vi "Get_CtrFile.vi"(8 "error in (no error)":errorcluster, 11 "IB_CtrFile in":refnum<class "IB_CtrFile.lvclass">) -> (0 "error out":errorcluster, 2 "parentTag":T1, 3 "IB_CtrFile out":refnum<class "IB_CtrFile.lvclass">)   [LabVIEW 2020, in "IB_CtrFile.lvclass"]
uses:
  <vilib>/AppBuilder/IB_Classes/Source/File/CtrFile/IB_CtrFile.lvclass
  <vilib>/AppBuilder/IB_Classes/Source/File/CtrFile/IB_CtrFile.lvclass/IB_CtrFile.ctl
  <vilib>/AppBuilder/IB_Classes/Source/File/IB_CtrFile.ctl
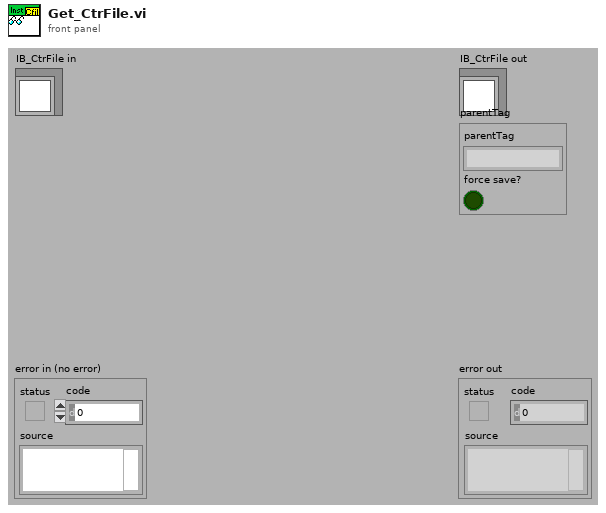
[diagram p1: front panel]
types:
  T1 = typedef "IB_CtrFile.ctl" = cluster{"parentTag":string, "force save?":bool}
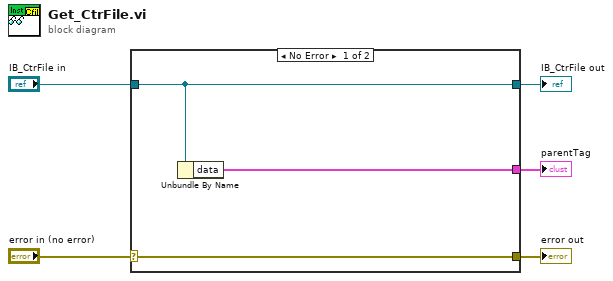
[diagram p0: block diagram]
diagram:
  n1 = case shown="No Error" "error in (no error)" {
    selector: "error in (no error)" -> [w8 w9]
    tunnel: [w8 w9] -> w4
    tunnel: [w7 w10] -> w2
    tunnel: "IB_CtrFile in" -> [w7 w10]
    tunnel: [w6 _] -> w1
    frame No Error {
      n2 = Unbundle By Name(w7) -> ("data"=w6:T1)
    }
    frame Error {
    }
  }
  "error out" <- w4
  "IB_CtrFile out" <- w2
  "parentTag" <- w1
